vi "UIMessage Callback.vi"(4 "Variant":variant, 5 "Event Data":cluster{"msg":refnum<k7>}, 6 "Control Ref":refnum<k7>, 7 "Event Common Data":T2) -> ()   [LabVIEW 2020, in "TSnax.lvlib" / "Engine.lvclass"]
uses:
  Engine.lvclass
  UIMsg.ctl
  Engine.lvclass/Engine.ctl
  UIMessage/UIMessage.lvclass
  TSnax.lvlib
panel:
  out "Code":T1
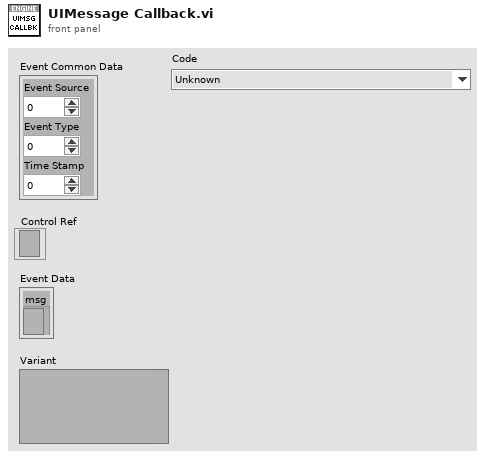
[diagram p1: front panel]
types:
  T1 = typedef "TSnax.lvlib/UIMsg.ctl" = enum16{"Unknown", "BreakOnUserRequest", "BreakOnBreakpoint", "BreakOnRunTimeError", "Trace", "TerminatingExecution", "AbortingExecution", "KillingExecutionThreads", "EndExecution", "ShutDownComplete", "StartExecution", "ProgressPercent", "ProgressText", "StartInteractiveExecution", "EndInteractiveExecution", "TerminatingInteractiveExecution", "TerminationCancelled", "ResumeFromBreak", "StartFileExecution", "EndFileExecution", "ShutDownCancelled", "LocalizationSettingChanged", "OpenWindows", "TileWindows", "CascadeWindows", "ReportChanged", "CloseWindows", "RefreshWindows", "ClientFileChanged", "DisplayReport", "ModelState_Initializing", "ModelState_Waiting", "ModelState_Identified", "ModelState_BeginTesting", "ModelState_TestingComplete", "ModelState_PostProcessingComplete", "ModelState_EnabledStateSet", "ReportLocationChanged", "GotoLocation", "PushUndoItem", "OutputMessages", "TypePaletteFileListChanged", "NonTerminatingThreadsArePreventingTermination", "ModelState_PostProcessing", "ReportCollectionChanged", "RuntimeError"}
  T2 = cluster{"Event Source":i32, "Event Type":u32, "Time Stamp":u32}
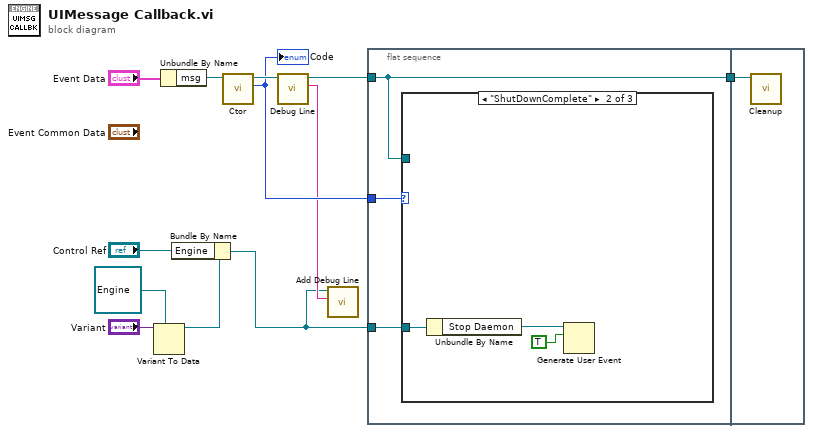
[diagram p0: block diagram]
diagram:
  n1 = Variant To Data(type=refnum<class "Engine.lvclass"> refnum ("TSnax.lvlib:Engine.lvclass"), Variant="Variant") -> (data=w2:refnum<class "Engine.lvclass">)  [unwired: 1 in, 1 out]
  n2 = Unbundle By Name("Event Data") -> ("msg"=w9:refnum<k7>)
  n3 = Bundle By Name(cluster=w2, "Engine"="Control Ref") -> (w1:refnum<class "Engine.lvclass">)
  n4 = call "Ctor.vi"("msg"=w9) -> ("Code"=w5:T1, "UIMessage out"=w8:refnum<class "UIMessage.lvclass">)  [unwired: 8 in, 1 out]
  "Code" <- w5
  n5 = call "Debug Line.vi"("UIMessage in"=w8) -> ("Debug Line"=w4:string, "UIMessage out"=w7:refnum<class "UIMessage.lvclass">)  [unwired: 9 in]
  n6 = call "Add Debug Line.vi"("Debug Line"=w4, "Engine in"=w1) -> ()  [unwired: 10 in]
  n7 = flat-sequence {
    tunnel: w7 -> [w15]
    tunnel: [w15] -> w6
    tunnel: w1 -> [w13]
    tunnel: w5 -> [w14]
    tunnel: w6 -> [w19]
    frame #0 {
      n8 = case shown="\"ShutDownComplete\"" w14 {
        tunnel: w15 -> [_ _ _]
        tunnel: w13 -> [_ w18 _]
        frame Default {
        }
        frame "ShutDownComplete" {
          n9 = Unbundle By Name(w18) -> ("Stop Daemon"=w17:refnum<user-event>)
          n10 = Generate User Event(user event=w17, event data cluster=TRUE ("event data")) -> ()  [unwired: 2 in, 2 out]
        }
        frame "ShutDownCancelled" {
        }
      }
    }
    frame #1 {
      n11 = call "Cleanup.vi"("UIMessage in"=w19) -> ()  [unwired: 10 in, 1 out]
    }
  }
